vi "Manual Waypoint Entry.vi"() -> (0 "WP List Out":T1[](array[typedef])=[{"Latitude"=2560.7253036, "Longitude"=4991.6912628}, {"Latitude"=2560.756671, "Longitude"=4991.7206508}, {"Latitude"=2560.7690244, "Longitude"=4991.7108402}, {"Latitude"=2560.7535018, "Longitude"=4991.6995968}, {"Latitude"=2560.7445954, "Longitude"=4991.6990676000005}, {"Latitude"=2560.7410314000003, "Longitude"=4991.7191292}, {"Latitude"=2560.7286606, "Longitude"=4991.7085092}, {"Latitude"=2560.7739798000002, "Longitude"=4991.6927112}] {"Longitude" format="%#_14g"; "Latitude" format="%#_14g"}, 1 "Nav Course Ending Location":T1 {"Longitude" format="%#_14g"; "Latitude" format="%#_14g"}, 2 "Nav Course Start Location":T1 {"Longitude" format="%#_14g"; "Latitude" format="%#_14g"})   [LabVIEW 2009]
uses:
  TypeDefs/Sensor TypeDefs/GPS Data.ctl
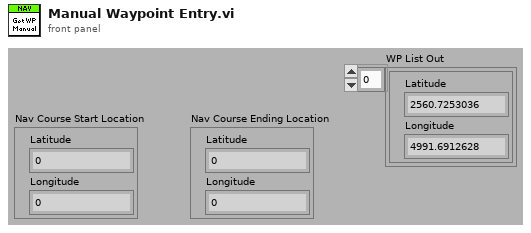
[diagram p1: front panel]
types:
  T1 = typedef "GPS Data.ctl" = cluster{"Latitude":dbl, "Longitude":dbl}
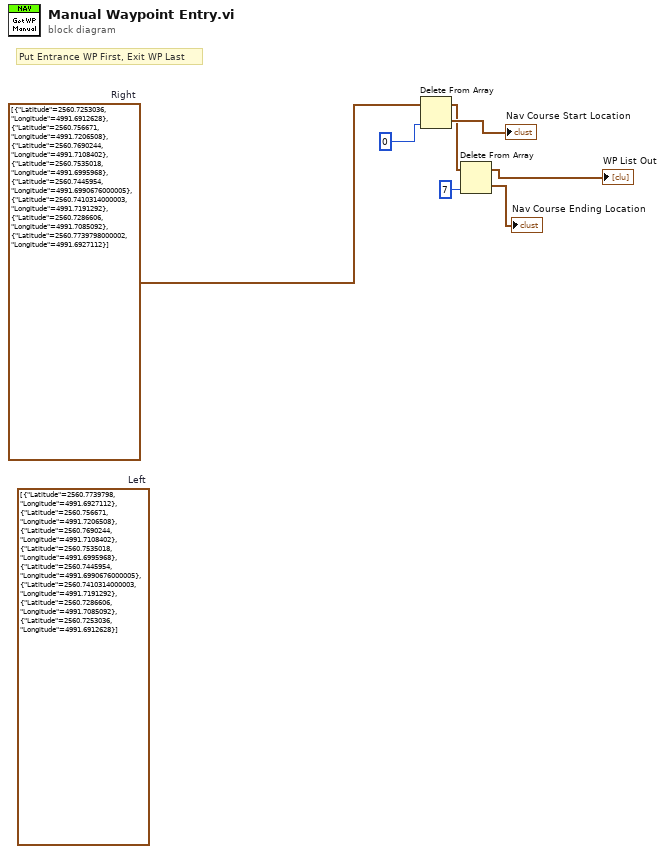
[diagram p0: block diagram]
diagram:
  (unwired) T1[] [{"Latitude"=2560.7739798, "Longitude"=4991.6927112}, {"Latitude"=2560.756671, "Longitude"=4991.7206508}, {"Latitude"=2560.7690244, "Longitude"=4991.7108402}, {"Latitude"=2560.7535018, "Longitude"=4991.6995968}, {"Latitude"=2560.7445954, "Longitude"=4991.6990676000005}, {"Latitude"=2560.7410314000003, "Longitude"=4991.7191292}, {"Latitude"=2560.7286606, "Longitude"=4991.7085092}, {"Latitude"=2560.7253036, "Longitude"=4991.6912628}]  # Left
  w1 = T1[] [{"Latitude"=2560.7253036, "Longitude"=4991.6912628}, {"Latitude"=2560.756671, "Longitude"=4991.7206508}, {"Latitude"=2560.7690244, "Longitude"=4991.7108402}, {"Latitude"=2560.7535018, "Longitude"=4991.6995968}, {"Latitude"=2560.7445954, "Longitude"=4991.6990676000005}, {"Latitude"=2560.7410314000003, "Longitude"=4991.7191292}, {"Latitude"=2560.7286606, "Longitude"=4991.7085092}, {"Latitude"=2560.7739798000002, "Longitude"=4991.6927112}]  # Right
  # "Put Entrance WP First, Exit WP Last"
  n1 = Delete From Array(array=w1, index=0) -> (deleted portion=→"Nav Course Start Location":T1, array with subset deleted=w5:T1[])  [unwired: 1 in]
  n2 = Delete From Array(array=w5, index=7) -> (deleted portion=→"Nav Course Ending Location":T1, array with subset deleted=→"WP List Out":T1[])  [unwired: 1 in]
